vi "ScopeTraceConnectionArray_FGV.vi"(7 "Command":enum16{"add", "get", "init"}(ring), 10 "connection ID":refnum<k5>, 11 "Nr.":i32) -> (2 "ID Array":refnum<k5>[](array[refnum]), 3 "connection ID out":refnum<k5>)   [LabVIEW 2013]
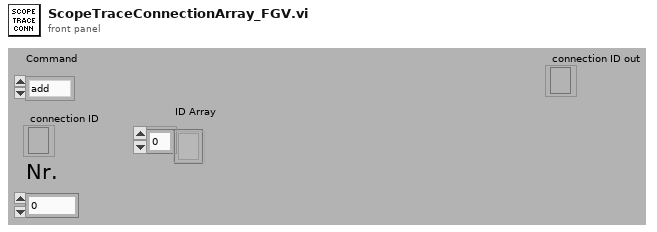
[diagram p1: front panel]
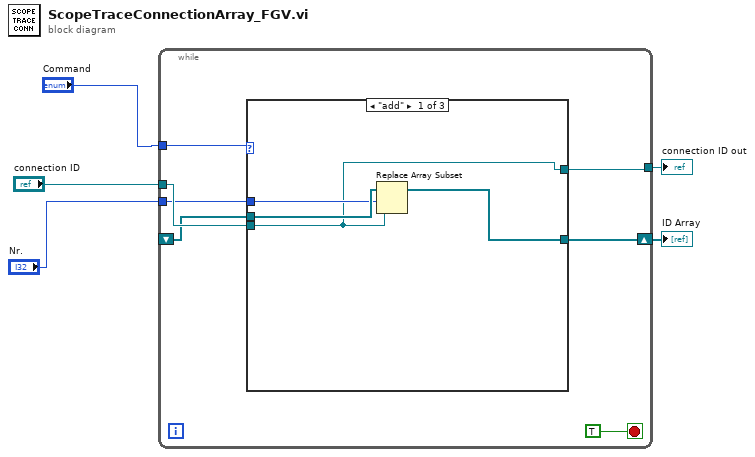
[diagram p0: block diagram]
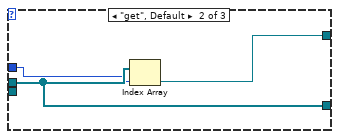
[diagram p2: hidden frame]
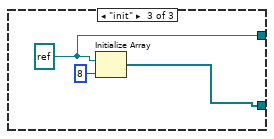
[diagram p3: hidden frame]
diagram:
  n1 = while {
    shift-right: [w9] -> w3
    shift-left: _ -> [w8]
    tunnel: "connection ID" -> [w10]
    tunnel: "Command" -> [w11]
    tunnel: "Nr." -> [w7]
    tunnel: [w6] -> w1
    stop <- TRUE stop-if-true
    n2 = case shown="\"add\"" w11 {
      tunnel: w10 -> [w13 _ _]
      tunnel: [w14 w19 w21] -> w9
      tunnel: w8 -> [w16 w19 _]
      tunnel: w7 -> [w15 w18 _]
      tunnel: [w13 w17 w20] -> w6
      frame "add" {
        n3 = Replace Array Subset(array=w16, new element=w13, index=w15) -> (w14:refnum<k5>[])
      }
      frame "get", Default {
        n4 = Index Array(array=w19, index=w18) -> (element=w17:refnum<k5>)
      }
      frame "init" {
        w20 = refnum<k5> refnum ("connection ID")
        n5 = Initialize Array(w20, 8 ("dimension size")) -> (w21:refnum<k5>[])
      }
    }
  }
  "ID Array" <- w3
  "connection ID out" <- w1
